vi "Main debug inline CD.vi"() -> ()   [LabVIEW 2021]
uses:
  <vilib>/NI VeriStand/Custom Device API/Hardware Interface Driver VI Operation.ctl
  <vilib>/NI VeriStand/Custom Device API/Custom Device API.lvlib
  SubVIs/states.ctl
  <vilib>/NI VeriStand/Custom Device API/Custom Device Item Ref.ctl
  <vilib>/Platform/TimedLoop/XDataNode/XDataNode.xnode
  <vilib>/Platform/TimedLoop/XDataNode/nitl_modes.ctl
  <vilib>/Platform/TimedLoop/XDataNode/XDNodeRunTimeDep.lvlib
  <vilib>/Platform/TimedLoop/XDataNode/wakeup.ctl
  <vilib>/Platform/TimedLoop/XDataNode/timing_clust.ctl
panel:
  in  "Period":i64=100
  in  "Stop Button":bool
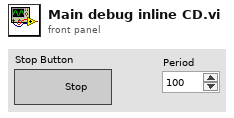
[diagram p1: front panel]
types:
  T1 = typedef "states.ctl" = enum16{"Init", "Start", "Update Global", "Read", "Write", "Shutdown"}
  T2 = typedef "XDNodeRunTimeDep.lvlib/timing_clust.ctl" = cluster{"Expected End [f-1]":u64, "Actual End [f-1]":u64, "Finished Late? [f-1]":bool, "Expected End [i-1]":u64, "Actual End [i-1]":u64, "Finished Late? [i-1]":bool, "Expected Start [i]":u64, "Actual Start [i]":u64, "Expected Start [f]":u64, "Actual Start [f]":u64, "Source Name":string, "Structure Name":string, "Period":i64, "Deadline":i64, "Offset":i64, "Start":i64, "Priority":i32, "Timeout":i32, "Mode":T3, "Wakeup Reason":T4, "Error":errorcluster, "Source Type":string, "Secondary Source Type":string, "Global End Time":u64, "Global Start Time":u64, "Frame Duration":u64, "Iteration Duration":u64, "Assigned CPU":i32, "I/O Scan Engine Mode":u32}
  T3 = typedef "XDNodeRunTimeDep.lvlib/nitl_modes.ctl" = enum32{"No Change", "Process missed periods, maintain original phase", "Discard missed periods, maintain original phase", "Process missed periods, ignore original phase", "Discard missed periods, ignore original phase"}
  T4 = typedef "XDNodeRunTimeDep.lvlib/wakeup.ctl" = enum32{"Normal", "Aborted", "Asynchronous wakeup", "Timing source error", "Timed loop error", "Timeout"}
  T5 = typedef "Custom Device API.lvlib/Custom Device Item Ref.ctl" = u64
  T6 = typedef "Custom Device API.lvlib/Hardware Interface Driver VI Operation.ctl" = enum16{"Initialize", "Start", "Read Data from HW", "Write Data to HW", "Close"}
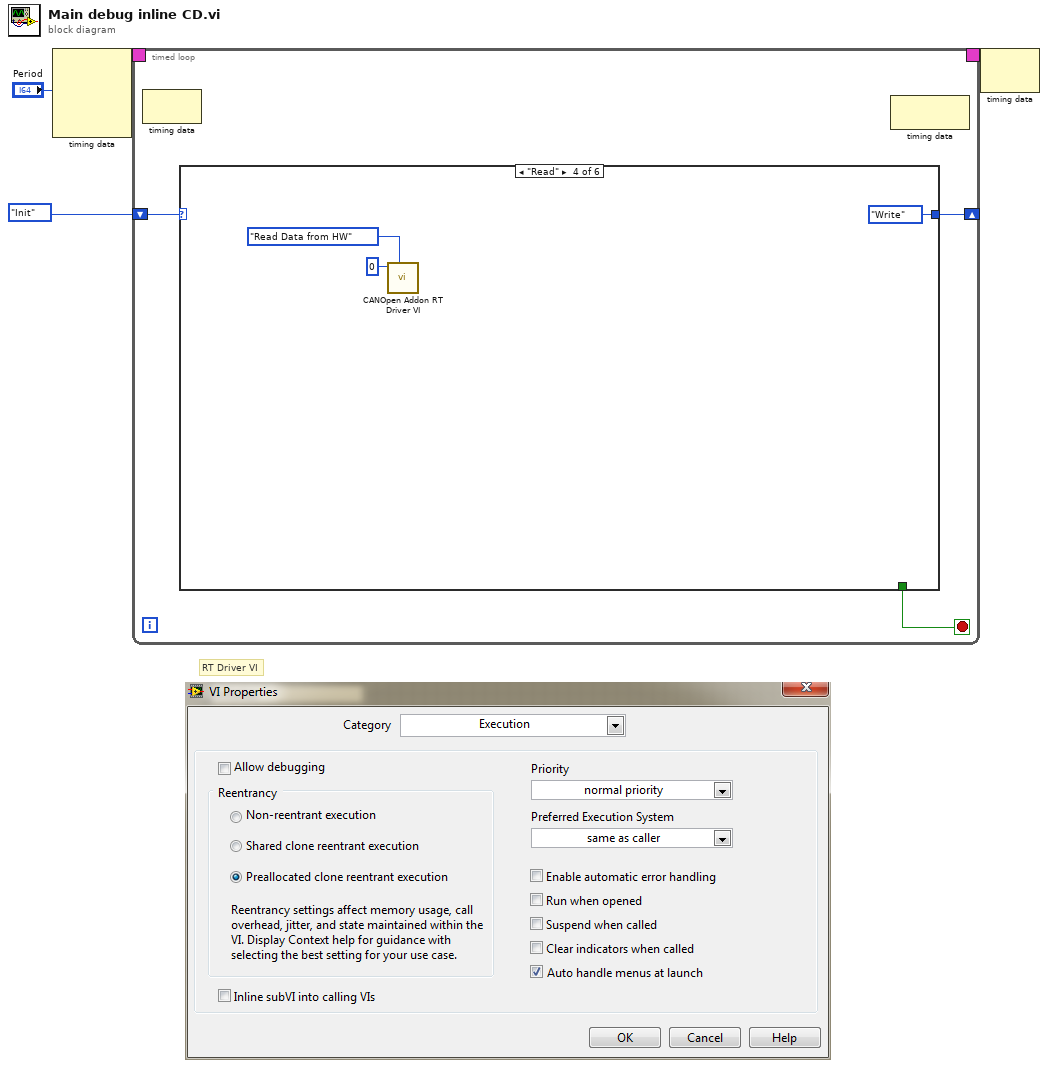
[diagram p0: block diagram]
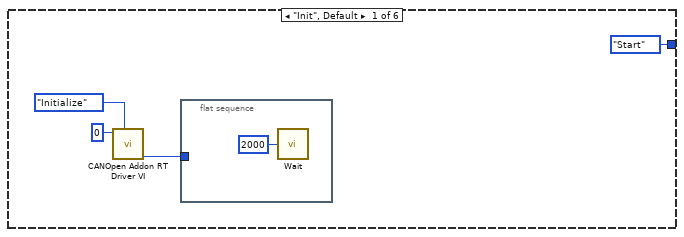
[diagram p2: hidden frame]
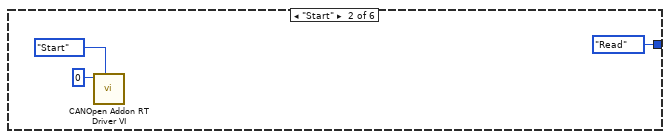
[diagram p3: hidden frame]
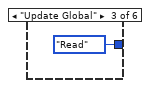
[diagram p4: hidden frame]
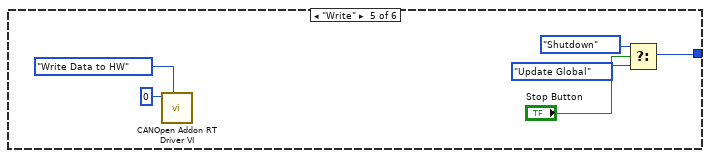
[diagram p5: hidden frame]
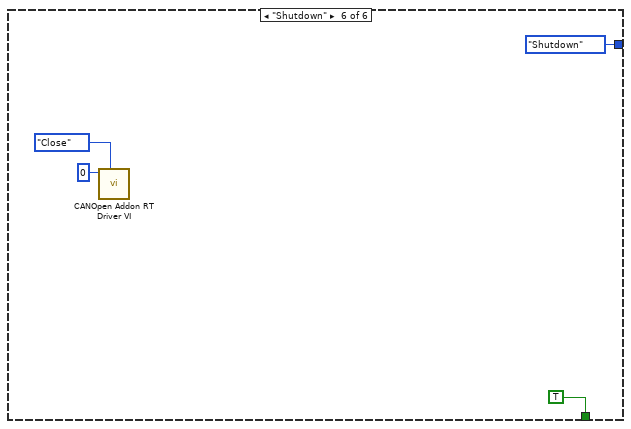
[diagram p6: hidden frame]
diagram:
  # "RT Driver VI"
  n1 = node-c288("Period") -> (w3:T2)  [unwired: 3 in]
  n2 = timed-loop {
    shift-right: [w6] -> _
    shift-left: states."Init" -> [w7]
    timing: w3 -> [_]
    timing-out: [_] -> w2
    stop <- w5 stop-if-true
    n3 = node-c288() -> ()  [unwired: 1 in, 1 out]
    n4 = case shown="\"Read\"" w7 {
      tunnel: [states."Start" states."Read" states."Read" states."Write" w25 states."Shutdown"] -> w6
      tunnel: [_ _ _ _ _ TRUE] -> w5
      frame "Init", Default {
        n5 = call "CANOpen Addon RT Driver VI.vi"("Operation"=Hardware_Interface_Driver_VI_Operation."Initialize", "Device Reference in"=T5 0) -> ("Error Code"=w10:i32)  [unwired: 9 in]
        n6 = flat-sequence {
          tunnel: w10 -> [_]
          frame #0 {
            n7 = call "Wait"("Count(mSec)"=u32 2000) -> ()  [unwired: 1 out]
          }
        }
      }
      frame "Start" {
        n8 = call "CANOpen Addon RT Driver VI.vi"("Operation"=Hardware_Interface_Driver_VI_Operation."Start", "Device Reference in"=T5 0) -> ()  [unwired: 9 in, 1 out]
      }
      frame "Update Global" {
      }
      frame "Read" {
        n9 = call "CANOpen Addon RT Driver VI.vi"("Operation"=Hardware_Interface_Driver_VI_Operation."Read Data from HW", "Device Reference in"=T5 0) -> ()  [unwired: 9 in, 1 out]
      }
      frame "Write" {
        n10 = call "CANOpen Addon RT Driver VI.vi"("Operation"=Hardware_Interface_Driver_VI_Operation."Write Data to HW", "Device Reference in"=T5 0) -> ()  [unwired: 9 in, 1 out]
        n11 = Select(t=states."Shutdown", s="Stop Button", f=states."Update Global") -> (s? t:f=w25:T1)
      }
      frame "Shutdown" {
        n12 = call "CANOpen Addon RT Driver VI.vi"("Operation"=Hardware_Interface_Driver_VI_Operation."Close", "Device Reference in"=T5 0) -> ()  [unwired: 9 in, 1 out]
      }
    }
    n13 = node-c288() -> ()  [unwired: 1 in, 1 out]
  }
  n14 = node-c288(w2) -> ()  [unwired: 1 out]
